vi "MGI Daemon.vi"(9 "Ignore Warnings? (F: Process Errors and Warnings)":bool, 10 "Log Dir":path=path "C:/Documents and Settings/All Users/Documents/Test Error Logs", 11 "ErrDialog In":refnum<class "MGI Error Reporter Dialog.lvclass">) -> (3 "ErrDialog Out":refnum<class "MGI Error Reporter Dialog.lvclass">)   [LabVIEW 2016, in "MGI Error Reporter Dialog.lvclass"]
doc: "This VI's Front Panel is the user interface dialog shown to the user. The block diagram code is minimal so that a child class may override it and redefine the look of the controls without having to modify the block diagram handling of the controls.\n\nAuthored by Shawn Walpole\nsupport@mooregoodideas.com\nwww.mooregoodideas.com\n\nCopyright (c) 2013, Moore Good Ideas, Inc.\n\nAll rights reserved.\n\nRedistribution and use in source and binary forms, with or without modification, are permitted provided that the following conditions are met:\n\n * Redistributions of source code must retain the above copyright notice, this list of conditions and the following disclaimer.\n * Redistributions in binary form must reproduce the above copyright notice, this list of conditions and the following disclaimer in the documentation and/or other materials provided with the distribution.\n * Neither the name of Moore Good Ideas, Inc. nor the names of its contributors may be used to endorse or promote products derived from this software without specific prior written permission.\n\nTHIS SOFTWARE IS PROVIDED BY THE COPYRIGHT HOLDERS AND CONTRIBUTORS \"AS IS\" AND ANY EXPRESS OR IMPLIED WARRANTIES, INCLUDING, BUT NOT LIMITED TO, THE IMPLIED WARRANTIES OF MERCHANTABILITY AND FITNESS FOR A PARTICULAR PURPOSE ARE DISCLAIMED. IN NO EVENT SHALL THE COPYRIGHT OWNER OR CONTRIBUTORS BE LIABLE FOR ANY DIRECT, INDIRECT, INCIDENTAL, SPECIAL, EXEMPLARY, OR CONSEQUENTIAL DAMAGES (INCLUDING, BUT NOT LIMITED TO, PROCUREMENT OF SUBSTITUTE GOODS OR SERVICES; LOSS OF USE, DATA, OR PROFITS; OR BUSINESS INTERRUPTION) HOWEVER CAUSED AND ON ANY THEORY OF LIABILITY, WHETHER IN CONTRACT, STRICT LIABILITY, OR TORT (INCLUDING NEGLIGENCE OR OTHERWISE) ARISING IN ANY WAY OUT OF THE USE OF THIS SOFTWARE, EVEN IF ADVISED OF THE POSSIBILITY OF SUCH DAMAGE."
uses:
  <userlib>/_MGI/Error Reporter/MGI Error Reporter Dialog/MGI Error Reporter Dialog.lvclass
  <userlib>/_MGI/Application Control/MGI Save & Restore Settings/MGI SRS Command Enum.ctl
  <userlib>/_MGI/Application Control/MGI VI Reference/MGI Current VI's Reference.vi
panel:
  in  "Clear History":bool
  in  "Error History LB":i32[](listbox) caption="History"
  out "Details Str":string caption="Details of selected error"
  in  "Call chain":u16(ring)
  out "Message Str":string caption="Message"
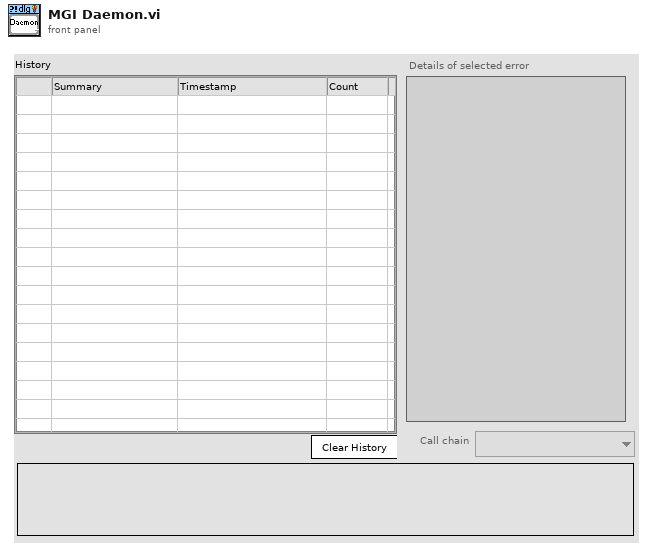
[diagram p1: front panel]
types:
  T1 = enum32{"Invalid", "Standard", "Closed", "Hidden", "Minimized", "Maximized"}
  T2 = typedef "MGI SRS Command Enum.ctl" = enum16{"Restore", "Save"}
  T3 = typedef "MGI Error Reporter Dialog.lvclass/MGI Dialog UI Refs Cluster.ctl" = cluster{"LB Ref":refnum<vi>, "Details Ref":refnum<vi>, "Caller Ring Ref":refnum<vi>, "Message Ref":refnum<vi>, "Clear Btn Ref":refnum<vi>}
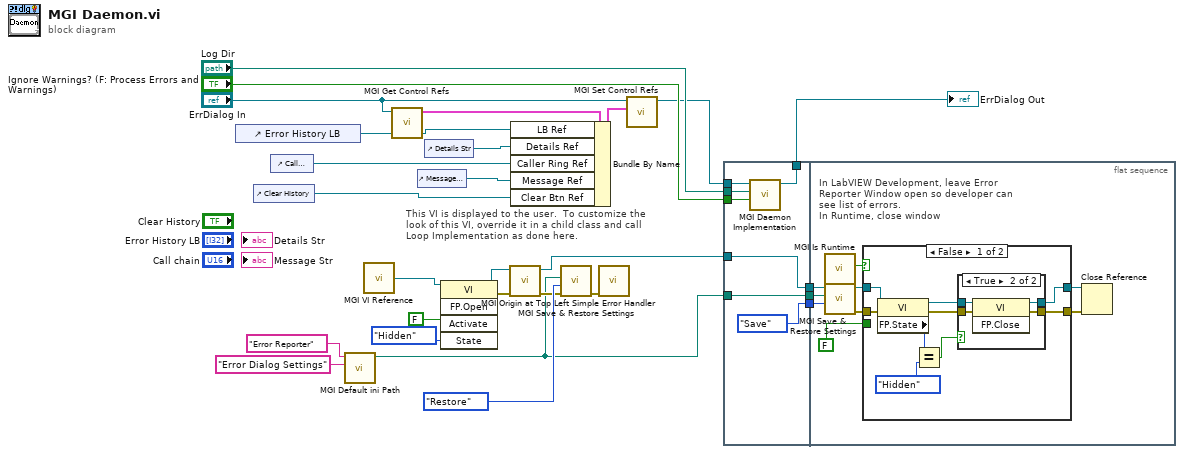
[diagram p0: block diagram]
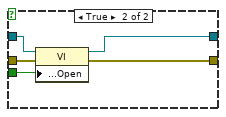
[diagram p3: hidden frame]
diagram:
  # "This VI is displayed to the user.  To customize the look of this VI, override it in a child class and call Loop Implementation as done here."
  n1 = control-ref of="Error History LB"() -> (w27:refnum<vi>)
  n2 = control-ref of="Clear History"() -> (w15:refnum<vi>)
  n3 = control-ref of="Call chain"() -> (w24:refnum<vi>)
  n4 = call <userlib>:"MGI Default ini Path.vi"("File Name (Caller's Prefix)"="Error Dialog Settings" ("string"), "Folder Name (Caller's Prefix)"="Error Reporter" ("string")) -> ("Path"=w2:path)  [unwired: 1 in, 8 out]
  n5 = call-poly <userlib>:"MGI VI Reference.vi"() -> ("Current VI's Reference"=w1:refnum<vi>)  [unwired: 1 out]
  n6 = call <userlib>:"MGI Get Control Refs.vi"("MGI Error Dialog.lvclass"="ErrDialog In") -> ("Refs"=w14:T3)  [unwired: 10 out]
  n7 = control-ref of="Message Str"() -> (w25:refnum<vi>)
  n8 = control-ref of="Details Str"() -> (w26:refnum<vi>)
  n9 = invoke class="VI" method="FP.Open"(reference=w1, "Activate"=FALSE ("Activate?"), "State"=T1."Hidden") -> (reference out=w4:refnum<vi>, error out=w7:errorcluster)  [unwired: 2 in, 3 out]
  n10 = call <userlib>:"MGI Origin at Top Left.vi"("Error In"=w7, "VI Reference In (Caller)"=w4) -> ("Error Out"=w6:errorcluster, "VI Reference Out"=w3:refnum<vi>)  [unwired: 7 out]
  n11 = Bundle By Name(cluster=w14, "LB Ref"=w27, "Details Ref"=w26, "Caller Ring Ref"=w24, "Message Ref"=w25, "Clear Btn Ref"=w15) -> (w12:T3)
  n12 = call <userlib>:"MGI Save & Restore Settings.vi"("Error In"=w6, "Command (Restore)"=MGI_SRS_Command_Enum."Restore", "Path"=w2) -> ("Error Out"=w5:errorcluster)  [unwired: 2 in, 6 out]
  n13 = call <vilib>:"Simple Error Handler.vi"("error in (no error)"=w5) -> ()  [unwired: 1 in, 8 out]
  n14 = call <userlib>:"MGI Set Control Refs.vi"("Refs"=w12, "MGI Error Handler In"="ErrDialog In") -> ("MGI Error Handler Out"=w11:refnum<class "MGI Error Reporter Dialog.lvclass">)  [unwired: 9 out]
  n15 = flat-sequence {
    tunnel: w2 -> [w34]
    tunnel: [w28] -> w22
    tunnel: [MGI_SRS_Command_Enum."Save" ("Command (Restore)")] -> w21
    tunnel: [w34] -> w20
    tunnel: w11 -> [w33]
    tunnel: [w32] -> w19
    tunnel: "Log Dir" -> [w31]
    tunnel: "Ignore Warnings? (F: Process Errors and Warnings)" -> [w30]
    tunnel: w3 -> [w28]
    tunnel: w22 -> [w43]
    tunnel: w21 -> [w42]
    tunnel: w20 -> [w41]
    frame #0 {
      n16 = call-dynamic "MGI Daemon Implementation.vi"("Ignore Warnings? (F: Process Errors and Warnings)"=w30, "Log Dir"=w31, "MGI Error Reporter Dialog In"=w33) -> ("MGI Error Reporter Out"=w32:refnum<class "MGI Error Reporter Dialog.lvclass">)  [unwired: 8 out]
    }
    frame #1 {
      # "In LabVIEW Development, leave Error Reporter Window open so developer can see list of errors.\nIn Runtime, close window"
      n17 = call <userlib>:"MGI Is Runtime.vi"() -> ("Run Time System?"=w40:bool)  [unwired: 7 out]
      n18 = call <userlib>:"MGI Save & Restore Settings.vi"("Command (Restore)"=w42, "Path"=w41, "VI Reference In (Caller)"=w43) -> ("Error Out"=w38:errorcluster, "VI Reference Out"=w39:refnum<vi>)  [unwired: 2 in, 5 out]
      n19 = case shown="False" w40 {
        tunnel: w39 -> [w52 w59]
        tunnel: w38 -> [w51 w63]
        tunnel: [w44 w62] -> w37
        tunnel: [w45 w61] -> w36
        tunnel: FALSE ("Front Panel Window:Open") -> [_ w60]
        frame False {
          n20 = property class="VI"(reference=w52, error in=w51) -> (reference out=w48:refnum<vi>, error out=w47:errorcluster, "FP.State"=w50:T1)
          n21 = Equal?(x=w50, y=T1."Hidden") -> (x = y?=w46:bool)
          n22 = case shown="True" w46 {
            tunnel: w48 -> [w54 w58]
            tunnel: w47 -> [w53 w57]
            tunnel: [w54 w56] -> w45
            tunnel: [w53 w55] -> w44
            frame False {
            }
            frame True {
              n23 = invoke class="VI" method="FP.Close"(reference=w58, error in=w57) -> (reference out=w56:refnum<vi>, error out=w55:errorcluster)  [unwired: 1 in, 1 out]
            }
          }
        }
        frame True {
          n24 = property class="VI"(reference=w59, error in=w63, "Front Panel.Open"=w60) -> (reference out=w61:refnum<vi>, error out=w62:errorcluster)
        }
      }
      n25 = Close Reference(reference=w36, error in (no error)=w37) -> ()  [unwired: 1 out]
    }
  }
  "ErrDialog Out" <- w19
